vi "Write Data (Dictionary).vi"(8 "error in (no error)":errorcluster, 10 "Data (Dictionary)":T1[](array[typedef]), 11 "Data Save":refnum<class "Data.lvclass">) -> (0 "error out":errorcluster, 3 "Data Save out":refnum<class "Data.lvclass">)   [LabVIEW 2016, in "Data.lvclass"]
uses:
  Data.lvclass
  Typedefs/Dictionary--cluster.ctl
  Data.lvclass/Data.ctl
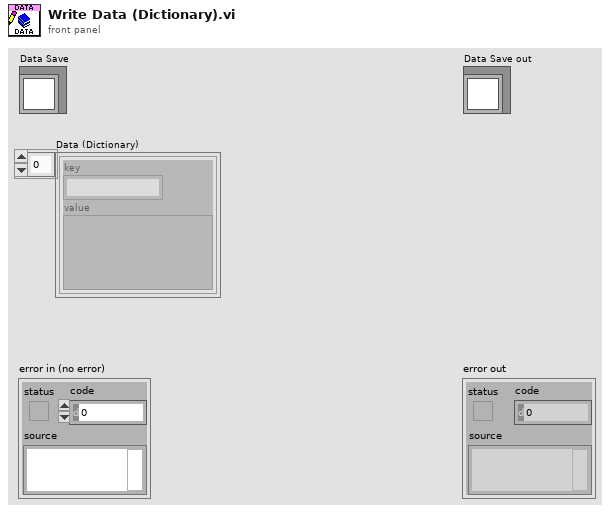
[diagram p1: front panel]
types:
  T1 = typedef "Data.lvclass/Dictionary--cluster.ctl" = cluster{"key":string, "value":variant}
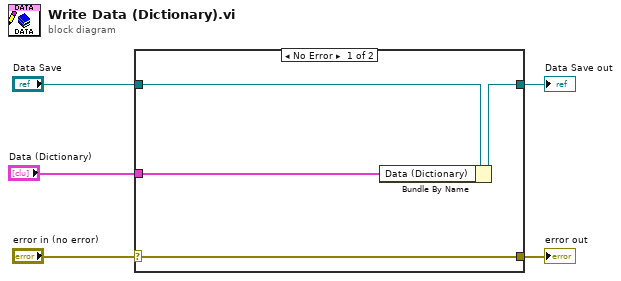
[diagram p0: block diagram]
diagram:
  n1 = case shown="No Error" "error in (no error)" {
    selector: "error in (no error)" -> [w9 w10]
    tunnel: [w9 w10] -> w4
    tunnel: [w6 w11] -> w2
    tunnel: "Data Save" -> [w8 w11]
    tunnel: "Data (Dictionary)" -> [w7 _]
    frame No Error {
      n2 = Bundle By Name(cluster=w8, "Data (Dictionary)"=w7) -> (w6:refnum<class "Data.lvclass">)
    }
    frame Error {
    }
  }
  "error out" <- w4
  "Data Save out" <- w2
